vi "Charging_Initialize.vi"(7 "file path (Rounded Square Wave Array)":path=path "C:/ATS Development/Code/Drivers/Charging/Rounded_Square_Wave_Array", 8 "error in (no error)":errorcluster, 10 "waveform settings":T1={"Frequency (40000 Hz)"=40000.0, "Offset (0 V)"=0.0, "Gain (3.7)"=3.7}, 11 "logical name (\"SampleFGen\")":refnum<k15> caption="instrument handle") -> (0 "error out":errorcluster, 1 "Arbitrary Waveform Handle [ARB]":i32, 3 "instrument handle out":refnum<k15>)   [LabVIEW 2010]
uses:
  <vilib>/Utility/file.llb/Read From Spreadsheet File (DBL).vi
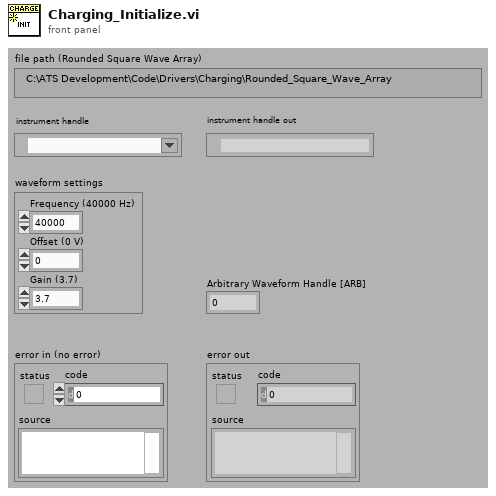
[diagram p1: front panel]
types:
  T1 = cluster{"Frequency (40000 Hz)":dbl, "Offset (0 V)":dbl, "Gain (3.7)":dbl}
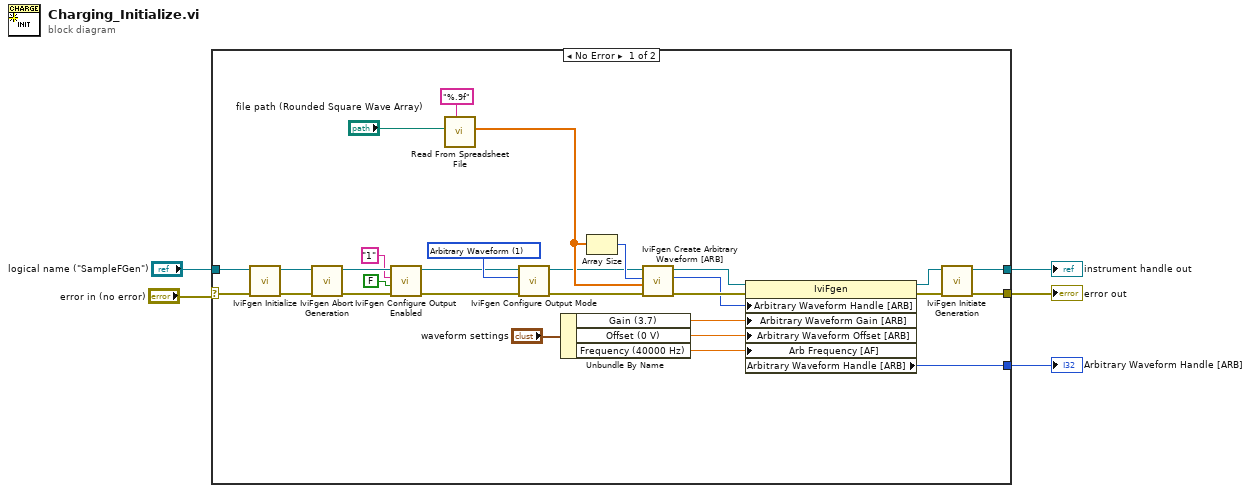
[diagram p0: block diagram]
diagram:
  n1 = case shown="No Error" "error in (no error)" {
    selector: "error in (no error)" -> [w32 w36]
    tunnel: [w6 w36] -> w4
    tunnel: "logical name (\"SampleFGen\")" -> [w17 w35]
    tunnel: [w23 _] -> w1
    tunnel: [w7 w35] -> w2
    frame No Error {
      w31 = 1 items=["Standard Function", "Arbitrary Waveform", "Arbitrary Sequence"] ("output mode (Standard Function)")
      n2 = call <vilib>:"IviFgen Initialize.vi"("error in (no error)"=w32, "logical name (\"SampleFGen\")"=w17) -> ("error out"=w18:errorcluster, "instrument handle out"=w16:refnum<k15>)  [unwired: 8 in]
      n3 = call <vilib>:"IviFgen Abort Generation.vi"("error in (no error)"=w18, "instrument handle"=w16) -> ("error out"=w9:errorcluster, "instrument handle out"=w10:refnum<k15>)  [unwired: 8 in]
      n4 = call <vilib>:"IviFgen Configure Output Enabled.vi"("error in (no error)"=w9, "channel enabled (True)"=FALSE, "channel name (\"CHANNEL1\")"="1" ("channel name (\"CHANNEL1\")"), "instrument handle"=w10) -> ("error out"=w15:errorcluster, "instrument handle out"=w14:refnum<k15>)  [unwired: 6 in]
      n5 = call-poly <vilib>:"Read From Spreadsheet File.vi"("format (%.3f)"="%.9f", "file path (dialog if empty)"="file path (Rounded Square Wave Array)") -> ("first row"=w29:dbl[])  [unwired: 5 in, 4 out]
      n6 = call <vilib>:"IviFgen Configure Output Mode.vi"("error in (no error)"=w15, "output mode (Standard Function)"=w31, "instrument handle"=w14) -> ("error out"=w11:errorcluster, "instrument handle out"=w12:refnum<k15>)  [unwired: 7 in]
      n7 = Unbundle By Name("waveform settings") -> ("Gain (3.7)"=w20:dbl, "Offset (0 V)"=w21:dbl, "Frequency (40000 Hz)"=w22:dbl)
      n8 = Array Size(array=w29) -> (size(s)=w30:i32)
      n9 = call <vilib>:"IviFgen Create Arbitrary Waveform [ARB].vi"("error in (no error)"=w11, "waveform data array (empty)"=w29, "waveform size (0)"=w30, "instrument handle"=w12) -> ("error out"=w26:errorcluster, "waveform handle"=w24:i32, "instrument handle out"=w27:refnum<k15>)  [unwired: 5 in]
      n10 = property class="IviFgen"(reference=w27, error in=w26, "Arbitrary Waveform Handle [ARB]"=w24, "Arbitrary Waveform Gain [ARB]"=w20, "Arbitrary Waveform Offset [ARB]"=w21, "Arb Frequency [AF]"=w22) -> (reference out=w28:refnum<k15>, error out=w25:errorcluster, "Arbitrary Waveform Handle [ARB]"=w23:i32)
      n11 = call <vilib>:"IviFgen Initiate Generation.vi"("error in (no error)"=w25, "instrument handle"=w28) -> ("error out"=w6:errorcluster, "instrument handle out"=w7:refnum<k15>)  [unwired: 8 in]
    }
    frame Error {
    }
  }
  "error out" <- w4
  "instrument handle out" <- w2
  "Arbitrary Waveform Handle [ARB]" <- w1
